vi "TemplateImageToBottomEdge (SubVI).vi"(7 "Pattern Match Settings":T5={"Algorithm"=2, "Number of Matches Requested"=1, "Minimum Match Score"=800.0, "SubPixel Accuracy"=TRUE, "Rotation Angle Ranges"=[{"Start"=0.0, "End"=0.0}], "Show Search Area"=FALSE, "Show Result"=TRUE} {"Rotation Angle Ranges"."End" format="%.1f"; "Rotation Angle Ranges"."Start" format="%.1f"; "Minimum Match Score" min=0 max=1000 format="%.2f"; "Number of Matches Requested" min=1; "Algorithm" items=["All", "Low Discrepancy Sampling", "Grayscale Value Pyramid", "Gradients Pyramid"]}, 8 "error in (no error)":errorcluster, 9 "Calibrated Image":T2, 10 "Search Rect":T4={"Left"=0, "Top"=0, "Right"=2147483647, "Bottom"=2147483647, "Rotation"=0.0} {"Rotation" format="%.2f"; "Left" scale=0.0..1024.0; "Right" scale=0.0..1024.0}, 11 "GenClassTagFlatRef in":refnum<vi>) -> (0 "error out":errorcluster, 1 "Pattern Match Position":dbl[](array[numeric]), 2 "ROI Descriptor after matches":T3, 3 "Refnum out":T2)   [LabVIEW 2016]
uses:
  <vilib>/vision/Image Controls.llb/IMAQ Image.ctl
  <vilib>/vision/NI_Vision_Development_Module.lvlib
  <resource>/objmgr/IMAQImage.rc
panel:
  in  "ROI Descriptor before matches":T1={"Global Rectangle"=[675, 567, 1751, 1642], "Contours"=[{"ID"=enum."External", "Type"=12, "Coordinates"=[1212, 1104, 85, 537, 0, 0]}]} {"Contours"."Type" items=["No Selection", "Point", "Line", "Rectangle", "Oval", "Polygon", "Freehand Region", "Annulus", "Unused2", "Unused3", "Broken Line", "Freehand Line", "Rotated Rectangle"]}
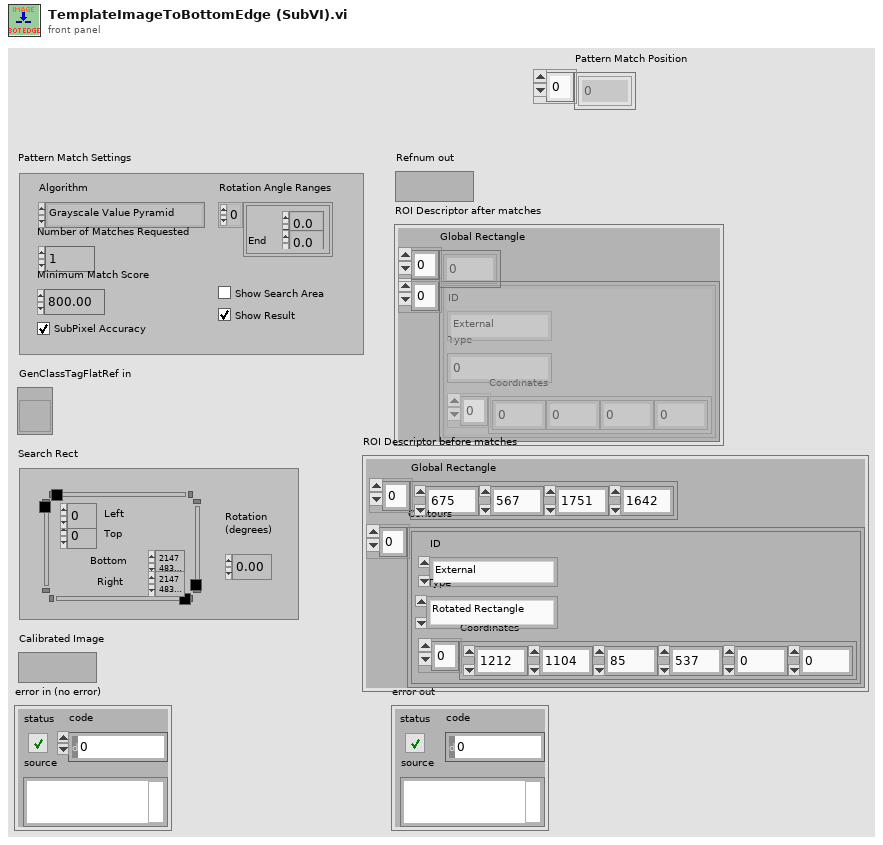
[diagram p1: front panel]
types:
  T1 = cluster{"Global Rectangle":i32[], "Contours":cluster{"ID":enum32{"External", "Internal"}, "Type":u32, "Coordinates":i32[]}[]}
  T2 = typedef "IMAQ Image.ctl" = refnum<image>
  T3 = cluster{"Global Rectangle":i32[], cluster{"ID":enum32{"External", "Internal"}, "Type":u32, "Coordinates":i32[]}[]}
  T4 = typedef "IMAQ Rectangle" = cluster{"Left":i32, "Top":i32, "Right":i32, "Bottom":i32, "Rotation":dbl}
  T5 = cluster{"Algorithm":i32, "Number of Matches Requested":i32, "Minimum Match Score":sgl, "SubPixel Accuracy":bool, "Rotation Angle Ranges":cluster{"Start":sgl, "End":sgl}[], "Show Search Area":bool, "Show Result":bool}
  T6 = cluster{"Left":i32, i32, "x":i32, "Bottom":i32, "Rotation":dbl}
  T7 = cluster{"Position":cluster{"x":sgl, "y":sgl}, "Angle":sgl, "Scale":sgl, "Score":sgl, "Bounding Box":cluster{"x":sgl, "y":sgl}[]}[]
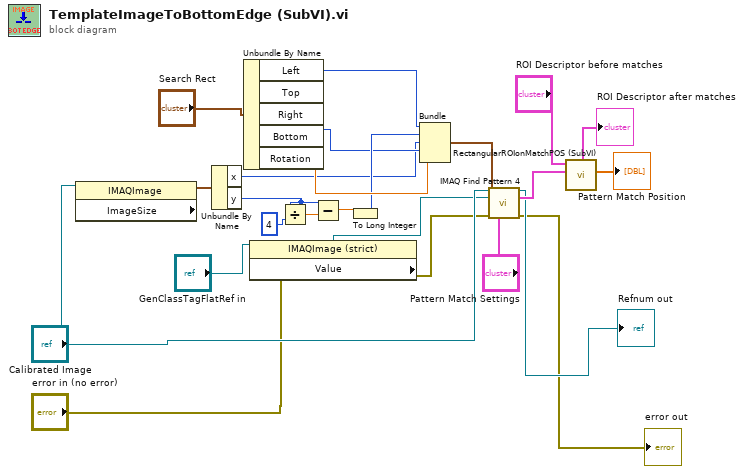
[diagram p0: block diagram]
diagram:
  n1 = property class="IMAQImage"(reference="Calibrated Image") -> ("ImageSize"=w20:cluster{"x":i32, "y":i32})  [unwired: 1 in, 2 out]
  n2 = Unbundle By Name(w20) -> ("x"=w4:i32, "y"=w8:i32)
  n3 = Unbundle By Name("Search Rect") -> ("Left"=w3:i32, "Bottom"=w5:i32, "Rotation"=w19:dbl)  [unwired: 2 out]
  n4 = property class="IMAQImage (strict)"(reference="GenClassTagFlatRef in") -> ("Value"=w11:T2)  [unwired: 1 in, 2 out]
  n5 = Divide(x=w8, y=4) -> (x/y=w9:dbl)
  n6 = Subtract(x=w8, y=w9) -> (x-y=w7:dbl)
  n7 = To Long Integer(number=w7) -> (32bit integer=w6:i32)
  n8 = Bundle("Left"=w3, w6, "x"=w4, "Bottom"=w5, "Rotation"=w19) -> (w23:T6)  [unwired: 1 in]
  n9 = call "IMAQ Find Pattern 4"("Image"="Calibrated Image", "Template"=w11, "Search Rect"=w23, "error in"="error in (no error)", "Settings"="Pattern Match Settings") -> ("Image Out"=→"Refnum out":T2, "Matches (pixel)"=w16:T7, "error out"=→"error out":errorcluster)  [unwired: 4 in, 4 out]
  n10 = call "RectangularROIonMatchPOS (SubVI).vi"("Matches (pixel)"=w16, "ROI Descriptor before matches"="ROI Descriptor before matches") -> ("Pattern Match Position"=→"Pattern Match Position":dbl[], "ROI Descriptor after matches"=→"ROI Descriptor after matches":T3)  [unwired: 8 in]
